vi "Load SG Parametersvi.vi"(8 "error in (no error)":errorcluster, 11 "Skyworks Spur Test in":refnum<class "Skyworks Spur Test.lvclass">) -> (0 "error out":errorcluster, 3 "Skyworks Spur Test out":refnum<class "Skyworks Spur Test.lvclass">)   [LabVIEW 2018, in "Skyworks Spur Test.lvlib" / "Skyworks Spur Test.lvclass"]
uses:
  Skyworks Spur Test.lvclass
  C:/Sequence Automation/Plugins/Measurement Interface.lvlibp/Measurement Interface.lvclass
  Skyworks Spur Test.lvclass/Skyworks Spur Test.ctl
  Write SG Parameters.vi
  Plugins/Measurement Interface.lvlibp/Private Methods/Measurement Parameters/Read Measurement Parameters.vi
  Plugins/String Database.lvlibp/String Database.lvclass
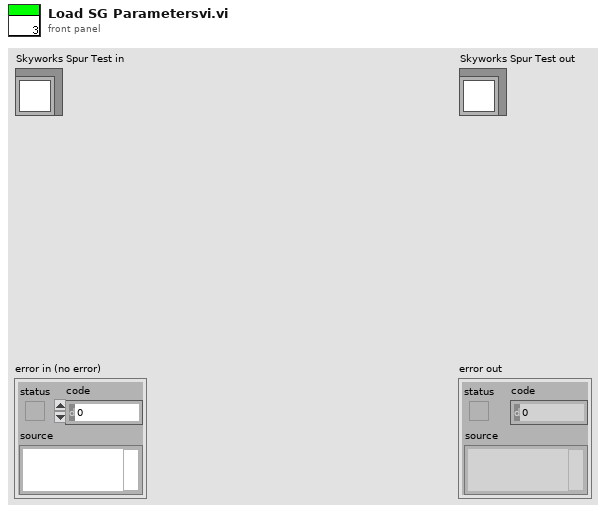
[diagram p1: front panel]
types:
  T1 = cluster{"Start Frequency":dbl, "Stop Frequency":dbl, "Delta":dbl}
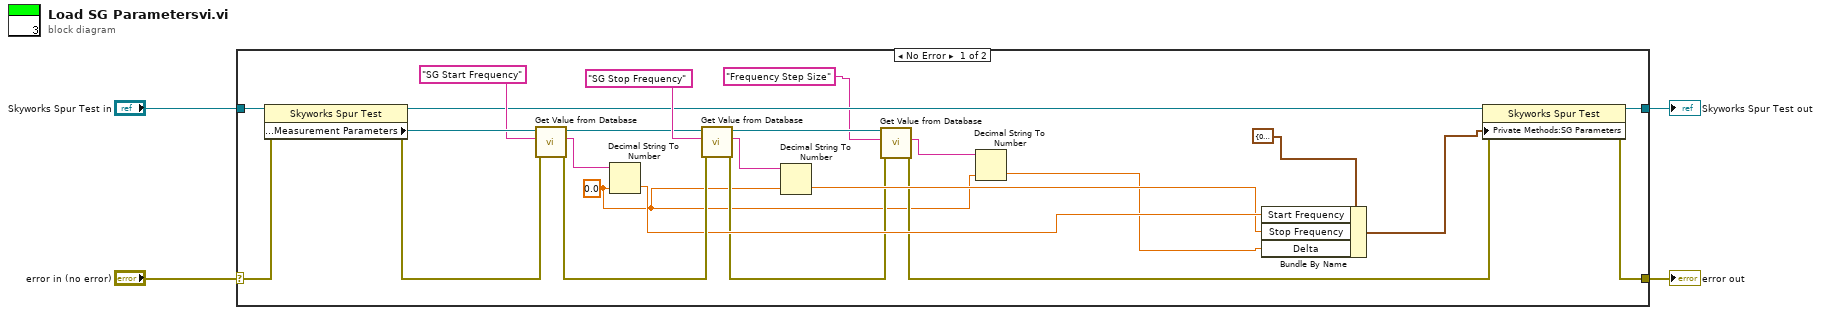
[diagram p0: block diagram]
diagram:
  n1 = case shown="No Error" "error in (no error)" {
    selector: "error in (no error)" -> [w28 w30]
    tunnel: [w21 w30] -> w3
    tunnel: [w19 w29] -> w1
    tunnel: "Skyworks Spur Test in" -> [w27 w29]
    frame No Error {
      w7 = 0.0 ("default (0 I32)")
      n2 = property class="Skyworks Spur Test"(reference=w27, error in=w28) -> (reference out=w20:refnum<class "Skyworks Spur Test.lvclass">, error out=w25:errorcluster, "Protected Methods:Measurement Parameters"=w26:refnum<class "String Database.lvclass">)
      n3 = call "Get Value from Database.vi"("error in (no error)"=w25, "Entry Name"="SG Start Frequency", "Message in"=w26) -> ("error out"=w17:errorcluster, "Entry Value"=w18:string, "Message out"=w22:refnum<class "String Database.lvclass">)  [unwired: 5 in, 1 out]
      n4 = Decimal String To Number(string=w18, default (0L)=w7) -> (number=w15:dbl)  [unwired: 1 in, 1 out]
      n5 = call "Get Value from Database.vi"("error in (no error)"=w17, "Entry Name"="SG Stop Frequency", "Message in"=w22) -> ("error out"=w11:errorcluster, "Entry Value"=w16:string, "Message out"=w12:refnum<class "String Database.lvclass">)  [unwired: 5 in, 1 out]
      n6 = Decimal String To Number(string=w16, default (0L)=w7) -> (number=w14:dbl)  [unwired: 1 in, 1 out]
      n7 = call "Get Value from Database.vi"("error in (no error)"=w11, "Entry Name"="Frequency Step Size", "Message in"=w12) -> ("error out"=w10:errorcluster, "Entry Value"=w8:string)  [unwired: 5 in, 2 out]
      n8 = Decimal String To Number(string=w8, default (0L)=w7) -> (number=w6:dbl)  [unwired: 1 in, 1 out]
      n9 = Bundle By Name(cluster=T1 {"Start Frequency"=0.0, "Stop Frequency"=0.0, "Delta"=0.0} ("SG Parameters"), "Start Frequency"=w15, "Stop Frequency"=w14, "Delta"=w6) -> (w5:T1)
      n10 = property class="Skyworks Spur Test"(reference=w20, error in=w10, "Private Methods:SG Parameters"=w5) -> (reference out=w19:refnum<class "Skyworks Spur Test.lvclass">, error out=w21:errorcluster)
    }
    frame Error {
    }
  }
  "error out" <- w3
  "Skyworks Spur Test out" <- w1
